vi "start_remote.vi"(8 "error in":errorcluster) -> (0 "error out":errorcluster, 3 "remoteQ":refnum<queue>)   [LabVIEW 2018]
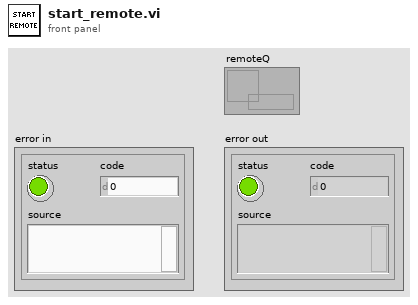
[diagram p1: front panel]
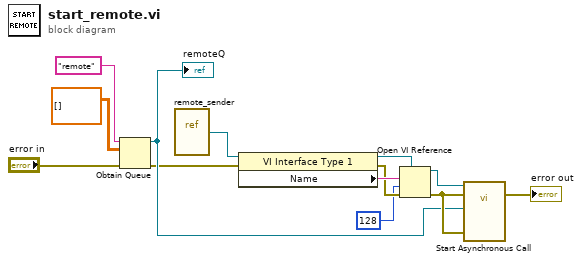
[diagram p0: block diagram]
diagram:
  n1 = Obtain Queue(name (unnamed)="remote", element data type=dbl[][] [] ("2D array"), error in (no error)="error in") -> (queue out=w3:refnum<queue>, error out=w2:errorcluster)  [unwired: 2 in, 1 out]
  "remoteQ" <- w3
  n2 = vi-ref "remote_sender.vi"() -> (w10:refnum<vi>)
  n3 = property class="VI Interface Type 1"(reference=w10, error in=w2) -> (reference out=w8:refnum<vi>, error out=w7:errorcluster, "Name"=w9:string)
  n4 = Open VI Reference(type specifier VI Refnum (for type only)=w8, vi path=w9, options=128, error in (no error)=w7) -> (vi reference=w6:refnum<vi>, error out=w4:errorcluster)  [unwired: 2 in]
  n5 = call-by-ref "Start Asynchronous Call"(reference=w6, error in=w4, "error in"=w4, "remote_queue"=w3) -> (error out=→"error out":errorcluster)  [unwired: 10 in, 1 out]
